vi "Gas line En-Type.vi"(4 "Gas Line Name String":string) -> (1 "Gas Line Name":T1)   [LabVIEW 2022 SP3]
uses:
  Anemometry/Anemometry Sub Vis/Controls/GMU Gas Line Name.ctl
  Anemometry/Anemometry Sub Vis/Globals/Trav_pos_global.vi
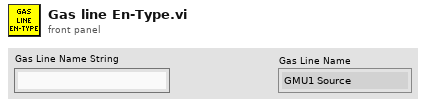
[diagram p1: front panel]
types:
  T1 = typedef "GMU Gas Line Name.ctl" = enum16{"GMU1 Source", "GMU2 Source", "GMU2 Calib", "CPP GRC-A", "CPP GRC-B"}
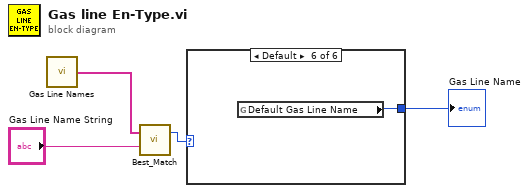
[diagram p0: block diagram]
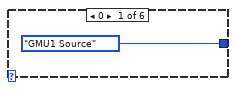
[diagram p2: hidden frame]
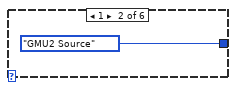
[diagram p3: hidden frame]
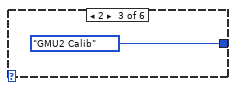
[diagram p4: hidden frame]
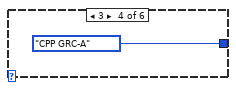
[diagram p5: hidden frame]
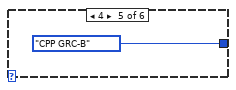
[diagram p6: hidden frame]
diagram:
  n1 = call "Gas Line Names.vi"() -> ("Gas line Names"=w3:string[])  [unwired: 5 in]
  n2 = call "Best_Match.vi"("Input String"="Gas Line Name String", "String Options"=w3) -> ("index of element"=w4:i32)  [unwired: 1 out]
  n3 = case shown="Default" w4 {
    tunnel: [GMU_Gas_Line_Name."GMU1 Source" ("Gas Line Name") GMU_Gas_Line_Name."GMU2 Source" ("Gas Line Name") GMU_Gas_Line_Name."GMU2 Calib" ("Gas Line Name") GMU_Gas_Line_Name."CPP GRC-A" ("Gas Line Name") GMU_Gas_Line_Name."CPP GRC-B" ("Gas Line Name") w10] -> w1
    frame 0 {
    }
    frame 1 {
    }
    frame 2 {
    }
    frame 3 {
    }
    frame 4 {
    }
    frame Default {
      n4 = global read "Trav_pos_global.vi" "Default Gas Line Name"() -> (w10:T1)
    }
  }
  "Gas Line Name" <- w1
